vi "BRig_Host_comm_webdav_connect.vi"() -> (0 "output_code":u8, 2 "output_Iconnected":bool, 3 "output_hSession":T1)   [LabVIEW 2014]
uses:
  <vilib>/WebDAVClient/Advanced/SessionHandle.ctl
  <vilib>/WebDAVClient/NI_WebDAV.lvlib
panel:
  out "error out":errorcluster
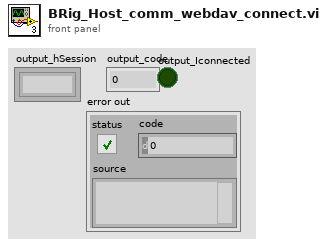
[diagram p1: front panel]
types:
  T1 = typedef "NI_WebDAV.lvlib/SessionHandle.ctl" = refnum<k1>
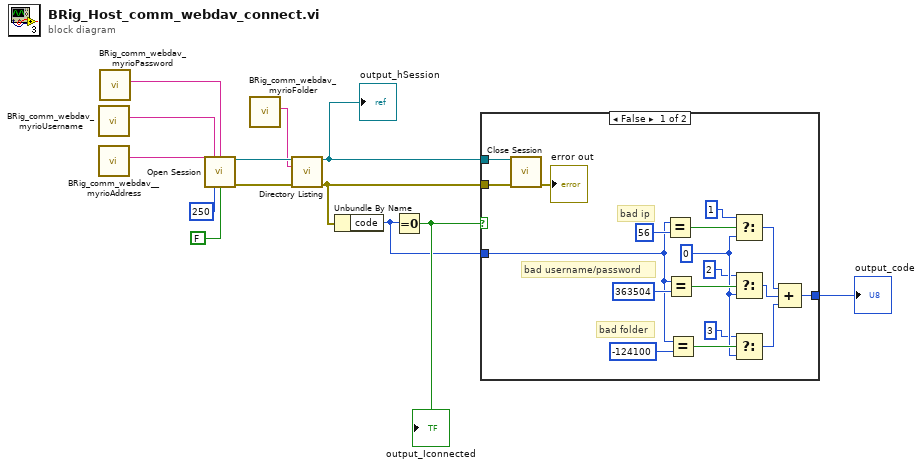
[diagram p0: block diagram]
diagram:
  n1 = call "BRig_comm_webdav_myrioUsername.vi"() -> ("output_myrioUsername"=w11:string)  [unwired: 11 in]
  n2 = call "BRig_comm_webdav__myrioAddress.vi"() -> ("output_myrioAddress"=w12:string)  [unwired: 11 in]
  n3 = call "BRig_comm_webdav_myrioPassword.vi"() -> ("output_myrioPassword"=w1:string)  [unwired: 11 in]
  n4 = call <vilib>:"Open Session.vi"("host uri prefix"=w12, "username"=w11, "password"=w1, "timeout ms"=250, "verify server?"=FALSE) -> ("session handle out"=w9:T1, "error out"=w8:errorcluster)  [unwired: 9 in]
  n5 = call "BRig_comm_webdav_myrioFolder.vi"() -> ("output_myrioFolder"=w7:string)  [unwired: 11 in]
  n6 = call <vilib>:"Directory Listing.vi"("session handle"=w9, "relative uri"=w7, "error in (no error)"=w8) -> ("session handle out"=w5:T1, "error out"=w4:errorcluster)  [unwired: 9 in, 2 out]
  "output_hSession" <- w5
  n7 = Unbundle By Name(w4) -> ("code"=w3:i32)
  n8 = Equal To 0?(x=w3) -> (x = 0?=w6:bool)
  "output_Iconnected" <- w6
  n9 = case shown="False" w6 {
    tunnel: w5 -> [w31 _]
    tunnel: w4 -> [w30 _]
    tunnel: w3 -> [w15 _]
    tunnel: [w14 _] -> w2
    frame False {
      w22 = u8 0
      # "bad folder"
      # "bad username/password"
      # "bad ip"
      n10 = call <vilib>:"Close Session.vi"("session handle"=w31, "error in (no error)"=w30) -> ("error out"=→"error out":errorcluster)  [unwired: 13 in]
      n11 = Equal?(x=w15, y=56) -> (x = y?=w25:bool)
      n12 = Equal?(x=w15, y=363504) -> (x = y?=w24:bool)
      n13 = Equal?(x=w15, y=-124100) -> (x = y?=w23:bool)
      n14 = Select(t=u8 1, s=w25, f=w22) -> (s? t:f=w16:u8)
      n15 = Select(t=u8 2, s=w24, f=w22) -> (s? t:f=w18:u8)
      n16 = Select(t=u8 3, s=w23, f=w22) -> (s? t:f=w17:u8)
      n17 = Compound Arithmetic op=ADD(w16, w18, w17) -> (w14:u8)
    }
    frame True {
    }
  }
  "output_code" <- w2
